vi "RunConversion.vi"(8 "error in (no error)":errorcluster, 11 "Model Driver in":refnum<class "Model Driver.lvclass">) -> (0 "error out":errorcluster, 3 "Model Driver out":refnum<class "Model Driver.lvclass">)   [LabVIEW 2023, in "Model Driver.lvclass"]
doc: "This method runs the ADC convertion VI."
uses:
  Model Driver.lvclass
  Multi-Channel ADC.vi
  Model Driver.lvclass/Model Driver.ctl
  Conversion/Conversion.lvclass
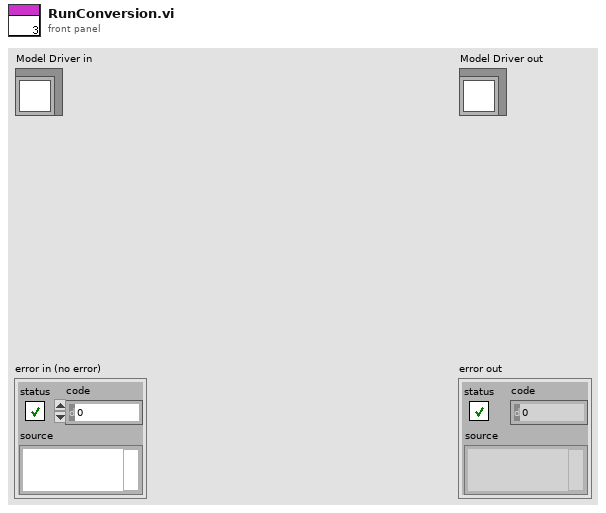
[diagram p1: front panel]
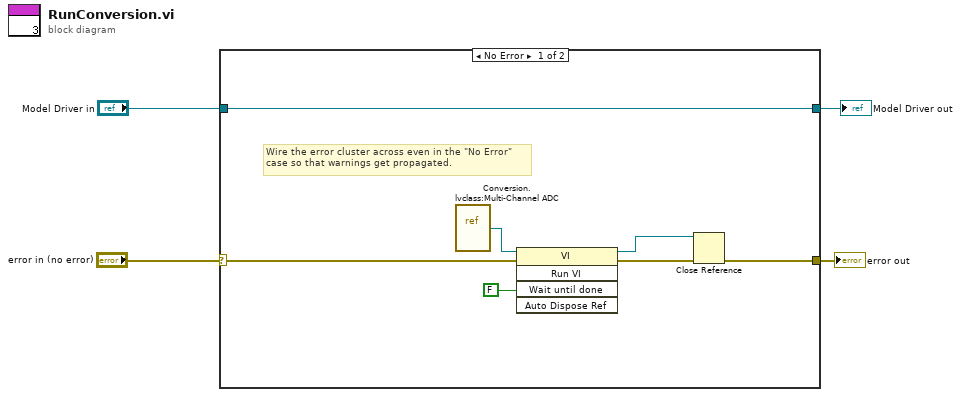
[diagram p0: block diagram]
diagram:
  n1 = case shown="No Error" "error in (no error)" {
    selector: "error in (no error)" -> [w8 w13]
    tunnel: [w6 w13] -> w3
    tunnel: [w11 w12] -> w1
    tunnel: "Model Driver in" -> [w11 w12]
    frame No Error {
      # "Wire the error cluster across even in the \"No Error\"\ncase so that warnings get propagated."
      n2 = vi-ref "Conversion.lvclass:Multi-Channel ADC.vi"() -> (w10:refnum<vi>)
      n3 = invoke class="VI" method="Run VI"(reference=w10, error in=w8, "Wait until done"=FALSE ("Wait Until Done")) -> (reference out=w5:refnum<vi>, error out=w7:errorcluster)  [unwired: 2 in, 3 out]
      n4 = Close Reference(reference=w5, error in (no error)=w7) -> (error out=w6:errorcluster)
    }
    frame Error {
    }
  }
  "error out" <- w3
  "Model Driver out" <- w1
